vi "Dyson_X682_Attachment_Provisioning_Tester_Ver 1.0.0.0.vi"() -> ()   [LabVIEW 2017]
uses:
  Ctrls/MainStep.ctl
  Ctrls/AllControls.ctl
  <vilib>/Utility/miscctls.llb/LVRowAndColumnTypeDef.ctl
  ComVIS/Files/Ini/WriteIniFiles_ByVarient.vi
panel:
  in  "Recipe":string(combo)
  in  "MES Status":bool
  in  "maintenance":bool
  in  "mode":enum32{"Production mode", "Engineering mode"}(tab)
  out "Fail resume":bool caption="TotalResult"
  out "Table":string[][](table)
  out "LogInfo":string caption="Log"
  in  "AlarmData":i32(listbox)=-1
  out "Device state":bool caption="TotalResult"
  out "CT":dbl format="%#_3f"
  in  "ProductID:":string
  in  "TestInfo":T1 {"Yield" format="%#_g%"}
  out "MES_Status":string
  out "TestMode":string
  in  "Stop":bool
  in  "Start":bool
  in  "Exit":bool
  in  "Login":bool
  out "Login_status":string="Operator:Operator"
  out "OpenStatus":string
  in  "error in (no error)":errorcluster caption="错误输入（无错误）"
  # "Dyson X682 Attachment Provisioning Tester  v1.0.0.0"
  # "Waiting Barcode scanning"
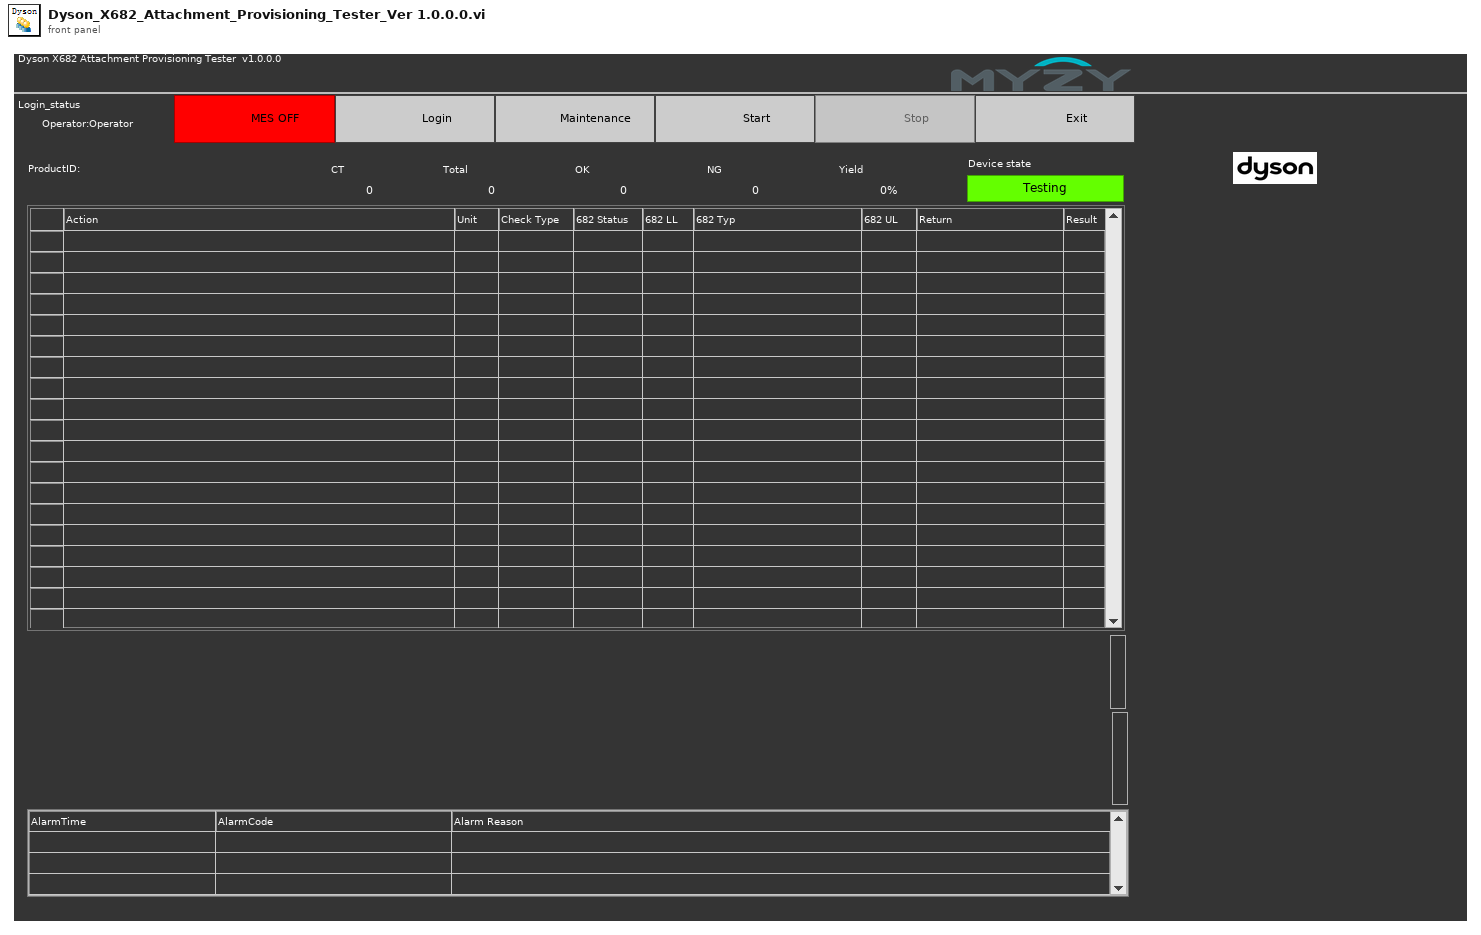
[diagram p1: front panel]
types:
  T1 = cluster{"Total":i32, "OK":i32, "NG":i32, "Yield":dbl}
  T2 = typedef "MainStep.ctl" = enum16{"Initialize", "ReadAllFiles", "ResetHardware", "Run", "Exit"}
  T3 = typedef "AllControls.ctl" = cluster{"MainVI":refnum<vi>, "AlarmInfo":refnum<vi>, "Log":refnum<vi>, "Current CT":refnum<vi>, "ProductID":refnum<vi>, "Device state":refnum<vi>, "MES":refnum<vi>, "mode":refnum<vi>, "TestInfo":refnum<vi>, "SubPnl":refnum<vi>, "Table":refnum<vi>, "MES bool":refnum<vi>, "TestMode":refnum<vi>, "Recipe":refnum<vi>, "Fail resume":refnum<vi>, "LogIn":refnum<vi>, "Start":refnum<vi>, "Maintenance":refnum<vi>, "Stop":refnum<vi>, "Exit":refnum<vi>}
  T4 = enum32{"Invalid", "Standard", "Closed", "Hidden", "Minimized", "Maximized"}
  T5 = enum16{"Ini", "Standby", "Running", "Engineering"}
  T6 = typedef "LVRowAndColumnTypeDef.ctl" = cluster{"Row":i32, "Column":i32}
  T7 = enum32{"invalid app kind", "Development System", "Run Time System", "Student Edition", "Embedded LabVIEW", "Evaluation", "Custom"}
  T8 = typedef "amc_Message Queue.ctl" = refnum<queue>
  T9 = typedef "HD Config.ctl" = cluster{" PC":cluster{"PC Address":u8[], "PC Port":i32}, "FCO":cluster{"COM":refnum<visa-resource-name>, "Baudrate":u32}, "DC Power ":cluster{"COM":refnum<visa-resource-name>, "Baudrate":u32}, "PW3336":cluster{"COM":refnum<visa-resource-name>, "Baudrate":u32}, "Lefoo":cluster{"COM":refnum<visa-resource-name>, "Baudrate":u32}, "AI Model":cluster{"COM":refnum<visa-resource-name>, "Baudrate":u32}, "DIPC":cluster{"COM":refnum<visa-resource-name>}, "RFID":cluster{"IP Address":string, "Port":u16, "Retry":u16}, "Motor":cluster{"COM":refnum<visa-resource-name>, "Baudrate":u32}, "Fail_resume_mode":bool, "GRR":bool}
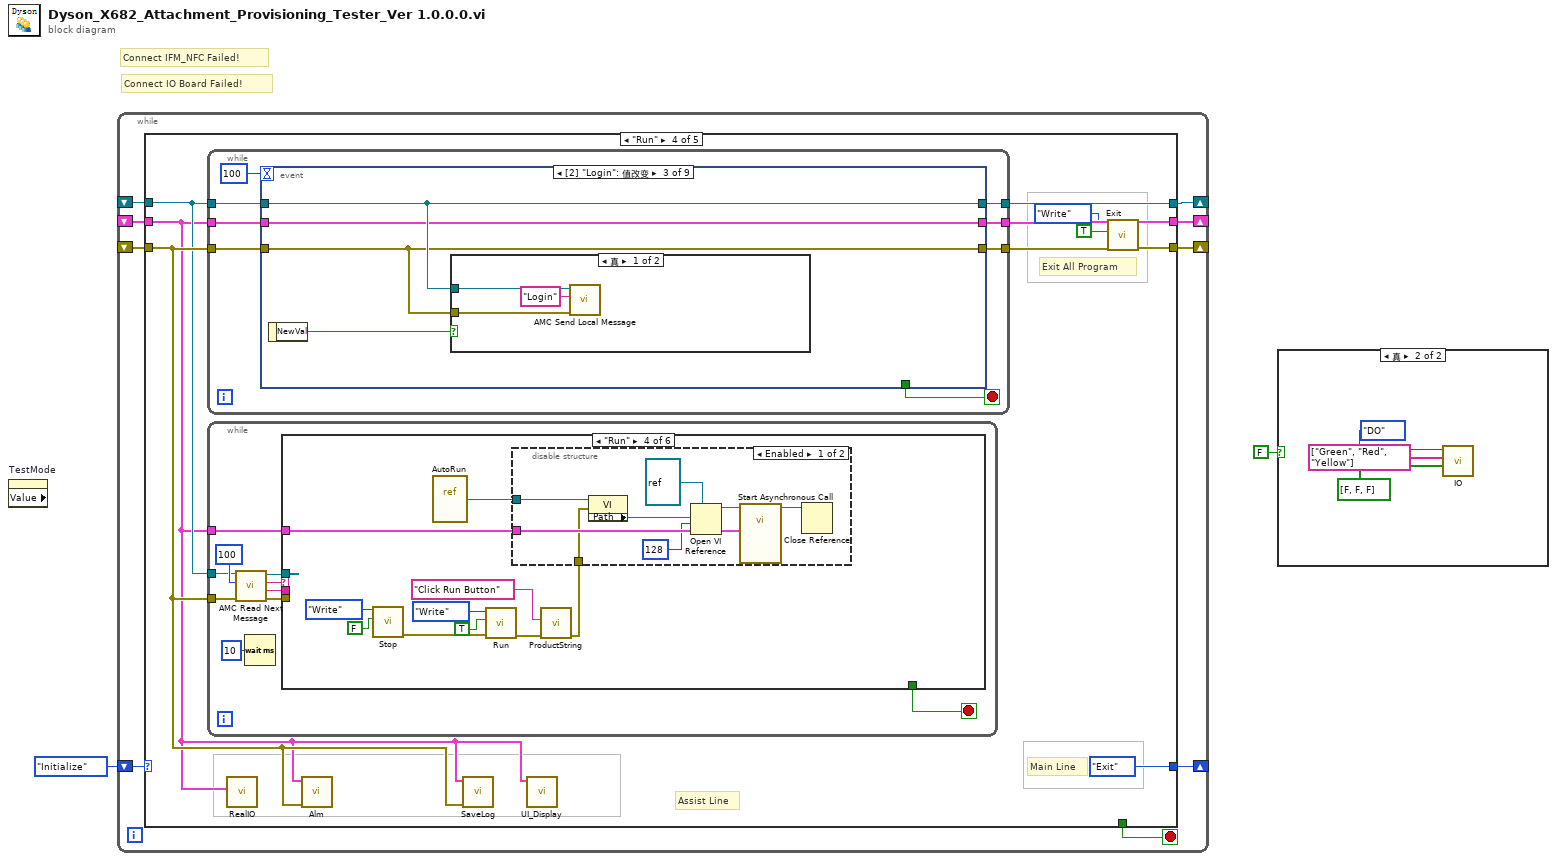
[diagram p0: block diagram]
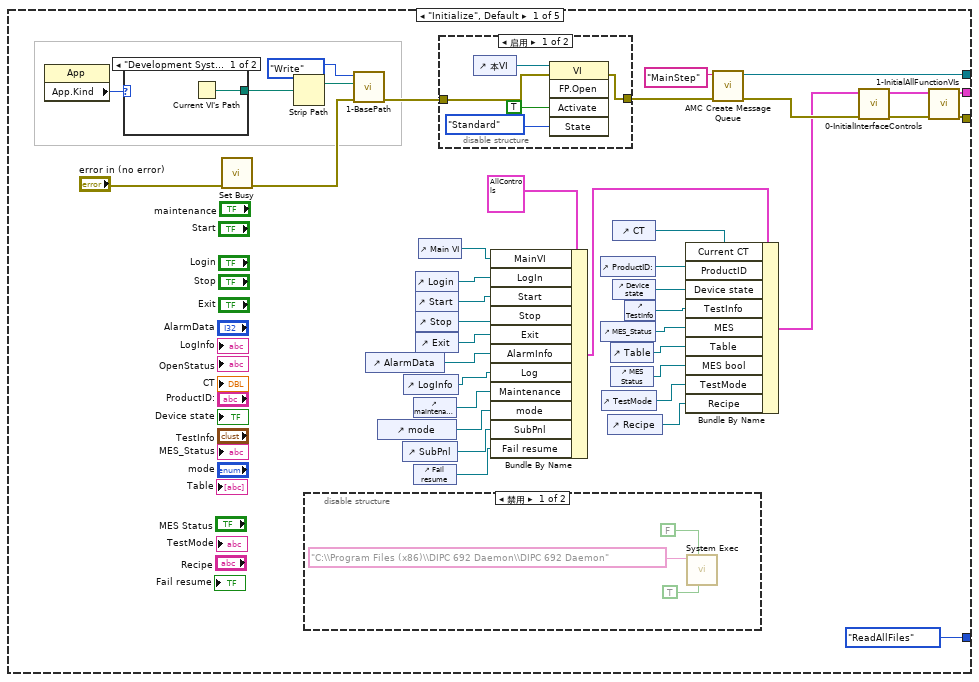
[diagram p3: hidden frame]
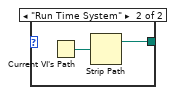
[diagram p6: hidden frame]
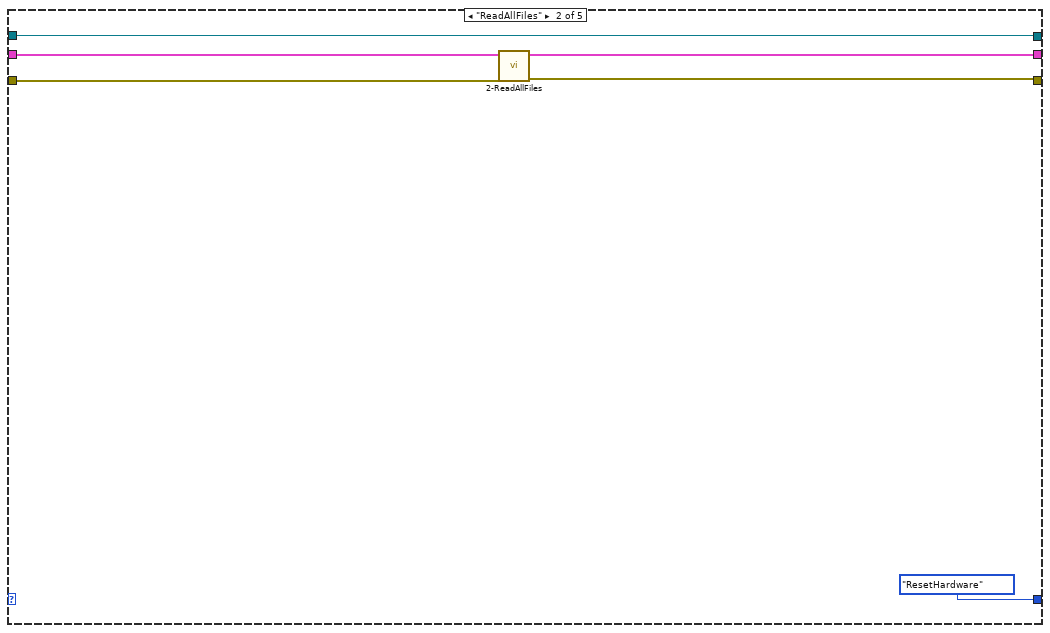
[diagram p7: hidden frame]
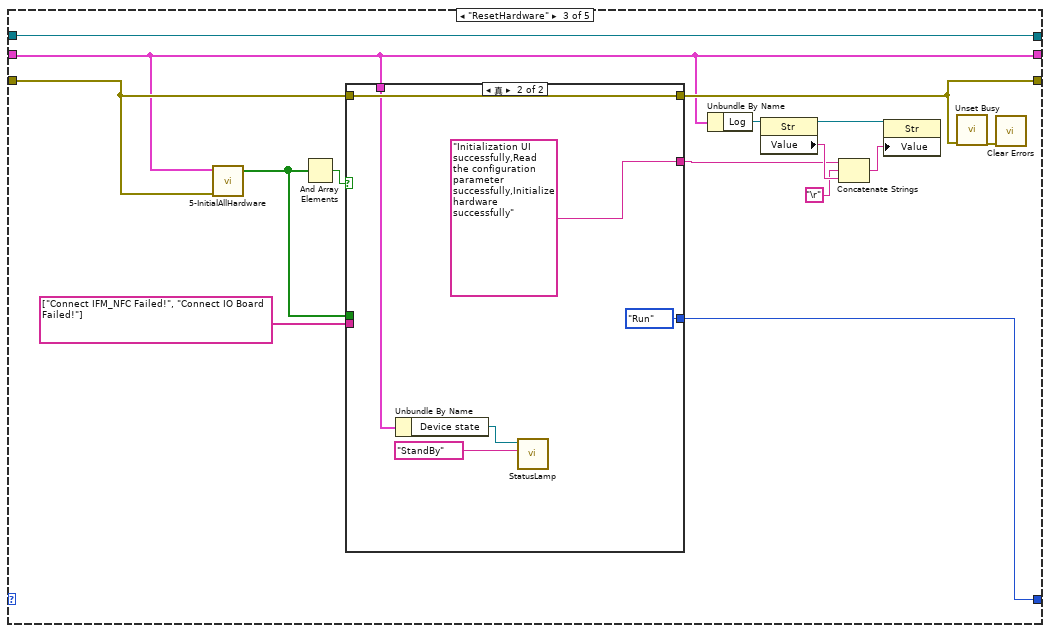
[diagram p8: hidden frame]
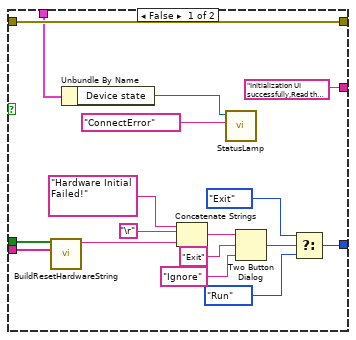
[diagram p9: hidden frame]
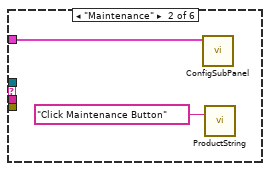
[diagram p11: hidden frame]
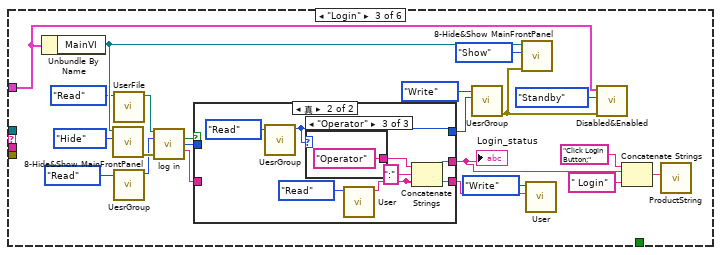
[diagram p12: hidden frame]
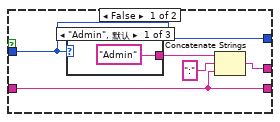
[diagram p13: hidden frame]
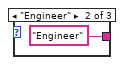
[diagram p14: hidden frame]
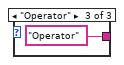
[diagram p15: hidden frame]
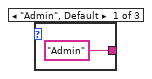
[diagram p16: hidden frame]
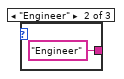
[diagram p17: hidden frame]
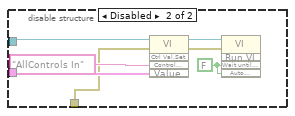
[diagram p18: hidden frame]
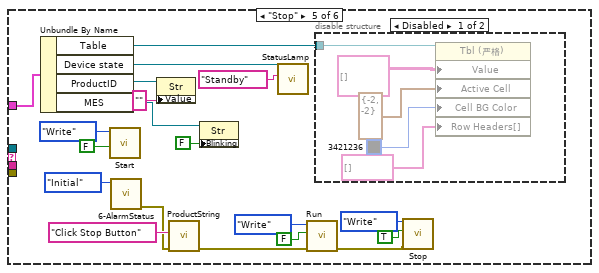
[diagram p19: hidden frame]
diagram:
  # "Connect IO Board Failed!"
  # "Connect IFM_NFC Failed!"
  n1 = property on="TestMode" class="Str" props=["Value"]() -> ()  [unwired: 2 in, 3 out]
  n2 = while {
    shift-right: [w10] -> _
    shift-left: MainStep."Initialize" -> [w11]
    shift-right: [w8] -> _
    shift-left: _ -> [w3]
    shift-right: [w6] -> _
    shift-left: _ -> [w4]
    shift-right: [w7] -> _
    shift-left: _ -> [w5]
    stop <- w9 stop-if-true
    n3 = case shown="\"Run\"" w11 {
      tunnel: [MainStep."ReadAllFiles" MainStep."ResetHardware" w83 MainStep."Exit" MainStep."Exit"] -> w10
      tunnel: [_ _ _ _ TRUE] -> w9
      tunnel: [w38 w63 w78 w110 w347] -> w8
      tunnel: [w46 w67 w82 w115 _] -> w7
      tunnel: [w39 w65 w76 w114 w345] -> w6
      tunnel: w5 -> [_ w67 w82 w108 w348]
      tunnel: w4 -> [_ w66 w76 w107 w345]
      tunnel: w3 -> [_ w64 w79 w109 w346]
      frame "Initialize", Default {
        n4 = property class="App"() -> ("App.Kind"=w50:T7)  [unwired: 2 in, 2 out]
        n5 = case shown="\"Development System\", 默认" w50 {
          tunnel: [w60 w61] -> w49
          frame "Development System", Default {
            n6 = Current VI's Path() -> (path=w60:path)
          }
          frame "Run Time System" {
            n7 = Current VI's Path() -> (path=w62:path)
            n8 = Strip Path(path=w62) -> (stripped path=w61:path)  [unwired: 1 out]
          }
        }
        n9 = call <vilib>:"Set Busy.vi"("error in (no error)"="error in (no error)") -> ("error out"=w18:errorcluster)  [unwired: 9 in, 1 out]
        n10 = Strip Path(path=w49) -> (stripped path=w19:path)  [unwired: 1 out]
        n11 = disable-structure shown="禁用" {
          frame Disabled {
            n12 = call <vilib>:"System Exec.vi"("run minimized? (F)"=TRUE, "wait until completion? (T)"=FALSE, "command line"="C:\\Program Files (x86)\\DIPC 692 Daemon\\DIPC 692 Daemon") -> ()  [unwired: 5 in, 4 out]
          }
          frame Enabled {
          }
        }
        n13 = call "1-BasePath.vi"("error in (no error)"=w18, "Path In"=w19, "Step"=enum16{"Initial", "Write", "Read"}."Write") -> ("error out"=w17:errorcluster)  [unwired: 7 in, 1 out]
        n14 = control-ref of="AlarmData"() -> (w44:refnum<vi>)
        n15 = control-ref of="mode"() -> (w25:refnum<vi>)
        n16 = control-ref of="SubPnl"() -> (w23:refnum<vi>)
        n17 = control-ref of="LogInfo"() -> (w43:refnum<vi>)
        n18 = control-ref of="maintenance"() -> (w24:refnum<vi>)
        n19 = control-ref of="Fail resume"() -> (w13:refnum<vi>)
        n20 = control-ref of="Login"() -> (w26:refnum<vi>)
        n21 = control-ref of="Start"() -> (w27:refnum<vi>)
        n22 = control-ref of="Stop"() -> (w28:refnum<vi>)
        n23 = control-ref of="Exit"() -> (w29:refnum<vi>)
        n24 = control-ref of="Main VI"() -> (w36:refnum<vi>)
        n25 = disable-structure shown="启用" {
          disable-tunnel: w17 -> [w56 w59]
          disable-tunnel: [w54 w59] -> w47
          frame Enabled {
            n26 = control-ref of="本VI"() -> (w58:refnum<vi>)
            n27 = invoke class="VI" method="FP.Open"(reference=w58, error in=w56, "Activate"=TRUE ("激活？"), "State"=T4."Standard" ("状态")) -> (error out=w54:errorcluster)  [unwired: 1 in, 4 out]
          }
          frame Disabled {
          }
        }
        n28 = Bundle By Name(cluster=T3 {"MainVI"=refnum, "AlarmInfo"=refnum, "Log"=refnum, "Current CT"=refnum, "ProductID"=refnum, "Device state"=refnum, "MES"=refnum, "mode"=refnum, "TestInfo"=refnum, "SubPnl"=refnum, "Table"=refnum, "MES bool"=refnum, "TestMode"=refnum, "Recipe"=refnum, "Fail resume"=refnum, "LogIn"=refnum, "Start"=refnum, "Maintenance"=refnum, "Stop"=refnum, "Exit"=refnum}, "MainVI"=w36, "LogIn"=w26, "Start"=w27, "Stop"=w28, "Exit"=w29, "AlarmInfo"=w44, "Log"=w43, "Maintenance"=w24, "mode"=w25, "SubPnl"=w23, "Fail resume"=w13) -> (w35:T3)
        n29 = control-ref of="ProductID:"() -> (w33:refnum<vi>)
        n30 = control-ref of="MES_Status"() -> (w30:refnum<vi>)
        n31 = control-ref of="TestMode"() -> (w15:refnum<vi>)
        n32 = control-ref of="Recipe"() -> (w14:refnum<vi>)
        n33 = control-ref of="Table"() -> (w21:refnum<vi>)
        n34 = control-ref of="MES Status"() -> (w16:refnum<vi>)
        n35 = control-ref of="CT"() -> (w32:refnum<vi>)
        n36 = control-ref of="Device state"() -> (w34:refnum<vi>)
        n37 = control-ref of="TestInfo"() -> (w31:refnum<vi>)
        n38 = Bundle By Name(cluster=w35, "Current CT"=w32, "ProductID"=w33, "Device state"=w34, "TestInfo"=w31, "MES"=w30, "Table"=w21, "MES bool"=w16, "TestMode"=w15, "Recipe"=w14) -> (w22:T3)
        n39 = call "AMC Create Message Queue.vi"("error in (no error)"=w47, "Message Queue Name"="MainStep" ("Message queue name (unnamed)")) -> ("error out"=w42:errorcluster, "Message Queue out"=w46:T8)  [unwired: 3 in, 5 out]
        n40 = call "0-InitialInterfaceControls.vi"("error in (no error)"=w42, "AllControls IN"=w22) -> ("error out"=w41:errorcluster, "AllControls Out"=w40:T3)  [unwired: 8 in]
        n41 = call "1-InitialAllFunctionVIs.vi"("error in (no error)"=w41, "AllControls IN"=w40) -> ("error out"=w38:errorcluster, "AllControls Out"=w39:T3)  [unwired: 8 in]
      }
      frame "ReadAllFiles" {
        n42 = call "2-ReadAllFiles.vi"("error in (no error)"=w64, "AllControls IN"=w66) -> ("error out"=w63:errorcluster, "AllControls Out"=w65:T3)  [unwired: 8 in]
      }
      frame "ResetHardware" {
        n43 = call "5-InitialAllHardware.vi"("error in (no error)"=w79, "AllControls IN"=w76) -> ("InitalResult"=w69:bool[])  [unwired: 9 in]
        n44 = And Array Elements(Boolean array=w69) -> (logical AND=w81:bool)
        n45 = case shown="真" w81 {
          tunnel: [w91 MainStep."Run"] -> w83
          tunnel: w79 -> [w100 w105]
          tunnel: string[] ["Connect IFM_NFC Failed!", "Connect IO Board Failed!"] -> [w89 _]
          tunnel: w69 -> [w90 _]
          tunnel: [w100 w105] -> w78
          tunnel: ["Initialization UI successfully,Read the configuration parameter successfully,Initialize hardware failure" ("值") "Initialization UI successfully,Read the configuration parameter successfully,Initialize hardware successfully" ("值")] -> w72
          tunnel: w76 -> [w84 w103]
          frame False {
            n46 = call "BuildResetHardwareString.vi"("String"=w89, "Error"=w90) -> ("DataOut"=w88:string)  [unwired: 9 in]
            n47 = Unbundle By Name(w84) -> ("Device state"=w85:refnum<vi>)
            n48 = Concatenate Strings("Hardware Initial Failed!" ("caption"), "\r", w88) -> (w98:string)
            n49 = call "StatusLamp.vi"("State"="ConnectError", "Boolean输入"=w85) -> ()  [unwired: 9 in, 1 out]
            n50 = Two Button Dialog(message=w98, 1:"Ignore" ("F按钮名称（“取消”）"), 2:"Exit" ("T按钮名称（“确定”）")) -> (T button?=w94:bool)
            n51 = Select(t=MainStep."Exit", s=w94, f=MainStep."Run") -> (s? t:f=w91:T2)
          }
          frame True {
            n52 = Unbundle By Name(w103) -> ("Device state"=w101:refnum<vi>)
            n53 = call "StatusLamp.vi"("State"="StandBy", "Boolean输入"=w101) -> ()  [unwired: 9 in, 1 out]
          }
        }
        n54 = Unbundle By Name(w76) -> ("Log"=w73:refnum<vi>)
        n55 = property class="Str"(reference=w73) -> (reference out=w71:refnum<vi>, "Value"=w75:string)  [unwired: 1 in, 1 out]
        n56 = Concatenate Strings(w72, "\r", w75) -> (w70:string)
        n57 = property class="Str"(reference=w71, "Value"=w70) -> ()  [unwired: 1 in, 2 out]
        n58 = call <vilib>:"Unset Busy.vi"("error in (no error)"=w78) -> ("error out"=w77:errorcluster)  [unwired: 10 in]
        n59 = call <vilib>:"Clear Errors.vi"("error in (no error)"=w77) -> ()  [unwired: 5 in, 2 out]
      }
      frame "Run" {
        # "Exit All Program"
        # "Assist Line"
        # "Main Line"
        n60 = while {
          tunnel: w108 -> [w227]
          tunnel: w107 -> [w226]
          tunnel: w109 -> [w225]
          tunnel: [w224] -> w115
          tunnel: [w223] -> w114
          tunnel: [w222] -> w111
          stop <- w221 stop-if-true
          n61 = event shown="[2] \"Login\": 值改变" {
            selector: _ -> [_ _ _ _ _ _ _ _ _]
            dyn-events: _ -> [_ _ _ _ _ _ _ _ _]
            timeout: 100 -> [_ _ _ _ _ _ _ _ _]
            tunnel: w227 -> [w230 w238 w263 w269 w281 w306 w320 w329 w336]
            tunnel: w226 -> [w229 w233 w261 w268 w279 w304 w318 w331 w341]
            tunnel: w225 -> [w228 w237 w262 w271 w280 w305 w319 w328 w337]
            tunnel: [w230 w238 w263 w269 w281 w306 w320 w329 w336] -> w224
            tunnel: [w229 w233 w261 w268 w279 w304 w318 w331 w341] -> w223
            tunnel: [w228 w237 w262 w271 w280 w305 w319 w328 w337] -> w222
            tunnel: [_ _ _ _ _ _ _ w327 w340] -> w221
            event Timeout {
              n62 = event-data() -> ()  [unwired: 1 in, 1 out]
            }
            event "Recipe": Value Change {
              n63 = event-data() -> ("OldVal"=w236:string, "NewVal"=w234:string)  [unwired: 1 in]
              n64 = Not Equal?(x=w236, y=w234) -> (x != y?=w235:bool)
              n65 = call "Run.vi"("Step"=enum16{"Initial", "Write", "Read"}."Read") -> ("Run Out"=w231:bool)  [unwired: 9 in, 1 out]
              n66 = case shown="假" w231 {
                tunnel: w235 -> [w241 _]
                tunnel: w234 -> [w240 _]
                tunnel: w233 -> [w239 _]
                frame False {
                  n67 = case shown="真" w241 {
                    tunnel: w240 -> [_ w255]
                    tunnel: w239 -> [_ w243]
                    frame False {
                    }
                    frame True {
                      w256 = cluster{"Recipe":string} {"Recipe"=""}  # Recipe
                      n68 = call "1-BasePath.vi"("Step"=enum16{"Initial", "Write", "Read"}."Read") -> ("Path Out"=w257:path)  [unwired: 9 in, 1 out]
                      n69 = call "ReadConfigandSetting.vi"("Recipe"=w255, "Path Out"=w257) -> ("TableData"=w244:string[][])  [unwired: 7 in, 2 out]
                      n70 = Bundle By Name(cluster=w256, "Recipe"=w255) -> (w254:cluster{"Recipe":string})
                      n71 = Build Path(base path=w257, name or relative path="data\\Recipe.ini") -> (appended path=w259:path)
                      n72 = Unbundle By Name(w243) -> ("Table"=w242:refnum<vi>)
                      n73 = call-poly "Read&WriteFile.vi"("Variant"=w254, "path"=w259) -> ()  [unwired: 9 in, 1 out]
                      n74 = Delete From Array(array=w244, length=1 ("长度"), index (row)=0 ("索引 (行)")) -> (deleted portion=w252:string[][], array with subset deleted=w250:string[][])  [unwired: 1 in]
                      n75 = call "Select_UUT_Table.vi"("all Title"=w252, "all Table"=w250) -> ("Title"=w251:string[], "Table"=w253:string[][])  [unwired: 8 in]
                      n76 = property class="Tbl (严格)"(reference=w242, "Value"=w253, "Column Headers[]"=w251, "Active Cell"=T6 {"Row"=-2, "Column"=-2} ("活动单元格:活动单元格"), "Cell BG Color"=u32 3421236, "Row Headers[]"=string[] [] ("Row Header Strings[]")) -> ()  [unwired: 1 in, 2 out]
                    }
                  }
                }
                frame True {
                }
              }
            }
            event "Login": Value Change {
              n77 = event-data() -> ("NewVal"=w264:bool)  [unwired: 1 in]
              n78 = case shown="真" w264 {
                tunnel: w263 -> [w267 _]
                tunnel: w262 -> [w266 _]
                frame True {
                  n79 = call "AMC Send Local Message.vi"("error in (no error)"=w266, "Message Name"="Login", "Message Queue in"=w267) -> ()  [unwired: 7 in, 2 out]
                }
                frame False {
                }
              }
            }
            event "maintenance": Value Change {
              n80 = event-data() -> ("NewVal"=w272:bool)  [unwired: 1 in]
              n81 = Unbundle By Name(w268) -> ("mode"=w270:refnum<vi>)
              n82 = case shown="真" w272 {
                tunnel: w270 -> [w278 _]
                tunnel: w269 -> [w275 _]
                tunnel: w268 -> [w274 _]
                frame True {
                  n83 = call "AMC Send Local Message.vi"("Message Name"="Maintenance", "Message Queue in"=w275) -> ()  [unwired: 8 in, 2 out]
                  n84 = property class="TabCtl (严格)"(reference=w278, "Value"=enum32{"Production mode", "Engineering mode"}."Engineering mode" ("值")) -> ()  [unwired: 1 in, 2 out]
                  n85 = call "Disabled&Enabled.vi"("Mode in"=T5."Engineering", "AllControls In"=w274) -> ()  [unwired: 9 in, 1 out]
                }
                frame False {
                }
              }
            }
            event "Start": Value Change {
              n86 = event-data() -> ("NewVal"=w282:bool)  [unwired: 1 in]
              n87 = case shown="真" w282 {
                tunnel: w281 -> [w287 _]
                tunnel: w280 -> [w286 _]
                tunnel: w279 -> [w283 _]
                frame True {
                  n88 = call "AMC Send Local Message.vi"("error in (no error)"=w286, "Message Name"="Run", "Message Queue in"=w287) -> ()  [unwired: 7 in, 2 out]
                  n89 = call "Disabled&Enabled.vi"("Mode in"=T5."Running", "AllControls In"=w283) -> ()  [unwired: 9 in, 1 out]
                }
                frame False {
                }
              }
            }
            event "MES Status": Value Change {
              n90 = event-data() -> ("NewVal"=w289:bool)  [unwired: 1 in]
              n91 = Unbundle By Name(w304) -> ("MES bool"=w297:refnum<vi>, "TestMode"=w288:refnum<vi>)
              n92 = call "HD_Config.vi"("Step"=enum16{"Initial", "Write", "Read"}."Read") -> ("HD Config out"=w296:T9)  [unwired: 9 in, 1 out]
              n93 = Unbundle By Name(w296) -> ("Fail_resume_mode"=w293:bool, "GRR"=w291:bool)
              n94 = Not(x=w289) -> (.not. x?=w295:bool)
              n95 = Or(x=w293, y=w295) -> (x .or. y?=w294:bool)
              n96 = case shown="假" w291 {
                tunnel: w294 -> [w308 _]
                tunnel: [w307 "GRR"] -> w292
                frame False {
                  n97 = case shown="真" w308 {
                    tunnel: ["Production" "Engineering"] -> w307
                    frame False {
                    }
                    frame True {
                    }
                  }
                }
                frame True {
                }
              }
              n98 = property class="Str"(reference=w288, "Value"=w292) -> ()  [unwired: 1 in, 2 out]
              n99 = Select(t="MES ON", s=w289, f="MES OFF") -> (s? t:f=w298:string)
              n100 = case shown="\"MES ON\", 默认" w298 {
                selector: w298 -> [w312 w315]
                tunnel: [TRUE FALSE] -> w300
                tunnel: [w312 w315] -> w301
                tunnel: [cluster{u32, u32}[] [{6618880, 6618880}] cluster{u32, u32}[] [{16711680, 16711680}]] -> w299
                frame "MES ON", Default {
                }
                frame "MES OFF" {
                }
              }
              n101 = property on="属性节点" class="Bool (严格)"(reference=w297, "Value"=w300, "Colors [4]"=w299, "BoolText.Text"=w301) -> ()  [unwired: 1 in, 2 out]
            }
            event "Stop": Value Change {
              n102 = event-data() -> ("NewVal"=w321:bool)  [unwired: 1 in]
              n103 = case shown="真" w321 {
                tunnel: w320 -> [w326 _]
                tunnel: w319 -> [w325 _]
                tunnel: w318 -> [w322 _]
                frame True {
                  n104 = call "AMC Send Local Message.vi"("error in (no error)"=w325, "Message Name"="Stop", "Message Queue in"=w326) -> ()  [unwired: 7 in, 2 out]
                  n105 = call "Disabled&Enabled.vi"("Mode in"=T5."Standby", "AllControls In"=w322) -> ()  [unwired: 9 in, 1 out]
                }
                frame False {
                }
              }
            }
            event "Exit": Value Change {
              n106 = event-data() -> ("NewVal"=w330:bool)  [unwired: 1 in]
              n107 = case shown="真" w330 {
                tunnel: w329 -> [_ w335]
                tunnel: w328 -> [_ w334]
                tunnel: [_ TRUE] -> w327
                frame False {
                }
                frame True {
                  n108 = call "AMC Send Local Message.vi"("error in (no error)"=w334, "Message Name"="Exit", "Message Queue in"=w335) -> ()  [unwired: 7 in, 2 out]
                }
              }
            }
            event Panel Close? {
              n109 = event-data() -> ()  [unwired: 1 in, 1 out]
              n110 = Two Button Dialog(message="Are you sure to Exit system?") -> (T button?=w339:bool)  [unwired: 2 in]
              n111 = case shown="假" w339 {
                selector: w339 -> [w343 w344]
                tunnel: [w343 w344] -> w340
                frame False {
                }
                frame True {
                }
              }
              n112 = Not(x=w340) -> (.not. x?=w342:bool)
              n113 = event-data("Discard?"=w342) -> ()  [unwired: 1 in, 1 out]
            }
          }
        }
        n114 = while {
          tunnel: w107 -> [w126]
          tunnel: w109 -> [w123]
          tunnel: w108 -> [w120]
          stop <- w117 stop-if-true
          n115 = call "AMC Read Next Message.vi"("error in (no error)"=w123, "timeout (1ms)"=100 ("Timeout"), "Message Queue in"=w120) -> ("error out"=w122:errorcluster, "Message Value"=w118:string, "Message Name"=w121:string, "Message Queue out"=w119:T8)  [unwired: 1 in, 4 out]
          n116 = Wait (ms)(milliseconds to wait=u32 10 ("毫秒倍数")) -> ()  [unwired: 1 out]
          n117 = case shown="\"Run\"" w121 {
            tunnel: w126 -> [_ w128 w136 w171 w211 _]
            tunnel: w122 -> [_ _ _ _ _ _]
            tunnel: [_ _ _ _ _ TRUE] -> w117
            tunnel: w119 -> [_ _ _ _ _ _]
            tunnel: w118 -> [_ _ _ _ _ _]
            frame "Null", Default {
            }
            frame "Maintenance" {
              n118 = call "ConfigSubPanel.vi"("AllControls"=w128) -> ()  [unwired: 11 in]
              n119 = call "ProductString.vi"("String"="Click Maintenance Button" ("值")) -> ()  [unwired: 10 in, 1 out]
            }
            frame "Login" {
              n120 = Unbundle By Name(w136) -> ("MainVI"=w149:refnum<vi>)
              n121 = call "8-Hide&Show MainFrontPanel.vi"("Hide&Show"=enum16{"Hide", "Show"}."Hide", "This VI"=w149) -> ("error out"=w147:errorcluster)  [unwired: 9 in]
              n122 = call "UserFile.vi"("Step"=enum16{"Initial", "Write", "Read"}."Read") -> ("UserPath out"=w146:path)  [unwired: 9 in, 1 out]
              n123 = call "UesrGroup.vi"("Step"=enum16{"Initial", "Write", "Read"}."Read") -> ("User group out"=w129:enum16{"Operator", "Engineer", "Admin"})  [unwired: 9 in, 1 out]
              n124 = call "log in.vi"("路径"=w146, "UserGroups in"=w129, "error in (no error)"=w147) -> ("Giveup?"=w144:bool, "UserGroups"=w143:enum16{"Operator", "Engineer", "Admin"}, "User"=w142:string)  [unwired: 8 in, 2 out]
              n125 = case shown="真" w144 {
                tunnel: [w152 w159] -> w138
                tunnel: [w153 w163] -> w132
                tunnel: [w151 w161] -> w140
                tunnel: w143 -> [w151 _]
                tunnel: w142 -> [w152 _]
                frame False {
                  n126 = case shown="\"Admin\", 默认" w151 {
                    tunnel: ["Admin" "Engineer" "Operator"] -> w155
                    frame "Admin", Default {
                    }
                    frame "Engineer" {
                    }
                    frame "Operator" {
                    }
                  }
                  n127 = Concatenate Strings(w155, ":" ("字符串"), w152) -> (w153:string)
                }
                frame True {
                  n128 = call "UesrGroup.vi"("Step"=enum16{"Initial", "Write", "Read"}."Read") -> ("User group out"=w161:enum16{"Operator", "Engineer", "Admin"})  [unwired: 9 in, 1 out]
                  n129 = case shown="\"Operator\"" w161 {
                    tunnel: ["Admin" "Engineer" "Operator"] -> w165
                    frame "Admin", Default {
                    }
                    frame "Engineer" {
                    }
                    frame "Operator" {
                    }
                  }
                  n130 = call "User.vi"("Step"=enum16{"Initial", "Write", "Read"}."Read") -> ("User out"=w159:string)  [unwired: 9 in, 1 out]
                  n131 = Concatenate Strings(w165, ":" ("字符串"), w159) -> (w163:string)
                }
              }
              "Login_status" <- w132
              n132 = call "UesrGroup.vi"("User group in"=w140, "Step"=enum16{"Initial", "Write", "Read"}."Write") -> ("错误输出"=w135:errorcluster)  [unwired: 8 in, 1 out]
              n133 = call "8-Hide&Show MainFrontPanel.vi"("error in (no error)"=w135, "Hide&Show"=enum16{"Hide", "Show"}."Show", "This VI"=w149) -> ()  [unwired: 8 in, 1 out]
              n134 = call "User.vi"("User in"=w138, "Step"=enum16{"Initial", "Write", "Read"}."Write") -> ()  [unwired: 8 in, 2 out]
              n135 = call "Disabled&Enabled.vi"("error in (no error)"=w135, "Mode in"=T5."Standby", "AllControls In"=w136) -> ()  [unwired: 8 in, 1 out]
              n136 = Concatenate Strings("Click Login Button;" ("String"), w132, " Login" ("字符串")) -> (w133:string)
              n137 = call "ProductString.vi"("String"=w133) -> ()  [unwired: 10 in, 1 out]
            }
            frame "Run" {
              n138 = call "Stop.vi"("Stop In"=FALSE ("AutoStopping In"), "Step"=enum16{"Initial", "Write", "Read"}."Write") -> ("error out"=w177:errorcluster)  [unwired: 8 in, 1 out]
              n139 = vi-ref "AutoRun.vi"() -> (w169:refnum<vi>)
              n140 = call "Run.vi"("error in (no error)"=w177, "Run In"=TRUE ("AutoRun In"), "Step"=enum16{"Initial", "Write", "Read"}."Write") -> ("error out"=w172:errorcluster)  [unwired: 7 in, 1 out]
              n141 = call "ProductString.vi"("error"=w172, "String"="Click Run Button" ("值")) -> ("error  out"=w170:errorcluster)  [unwired: 9 in]
              n142 = disable-structure shown="Enabled" {
                disable-tunnel: w171 -> [w183 w189]
                disable-tunnel: w170 -> [w181 w187]
                disable-tunnel: w169 -> [w180 w188]
                frame Enabled {
                  n143 = property class="VI"(reference=w180, error in=w181) -> ("Path"=w186:path)  [unwired: 2 out]
                  n144 = Open VI Reference(type specifier VI Refnum (for type only)=refnum<vi> refnum ("application reference (local)"), vi path=w186, options=128) -> (vi reference=w184:refnum<vi>)  [unwired: 3 in, 1 out]
                  n145 = call-by-ref "Start Asynchronous Call"(reference=w184, "AllControls In"=w183) -> (reference out=w182:refnum<vi>)  [unwired: 12 in, 1 out]
                  n146 = Close Reference(reference=w182) -> ()  [unwired: 1 in, 1 out]
                }
                frame Disabled {
                  w190 = FALSE ("Wait Until Done")
                  n147 = invoke class="VI" method="Ctrl Val.Set"(reference=w188, error in=w187, "Control Name"="AllControls In", "Value"=w189) -> (reference out=w192:refnum<vi>, error out=w193:errorcluster)  [unwired: 1 in, 3 out]
                  n148 = invoke class="VI" method="Run VI"(reference=w192, error in=w193, "Wait until done"=w190, "Auto Dispose Ref"=w190) -> ()  [unwired: 1 in, 5 out]
                }
              }
            }
            frame "Stop" {
              n149 = Unbundle By Name(w211) -> ("Table"=w205:refnum<vi>, "Device state"=w208:refnum<vi>, "ProductID"=w210:refnum<vi>, "MES"=w203:refnum<vi>)
              n150 = call "Start.vi"("Start In"=FALSE, "Step"=enum16{"Initial", "Write", "Read"}."Write") -> ()  [unwired: 8 in, 2 out]
              n151 = call "6-AlarmStatus.vi"("Step"=enum16{"Initial", "Write", "Read"}."Initial") -> ("error out"=w204:errorcluster)  [unwired: 9 in, 1 out]
              n152 = property class="Str"(reference=w210, "Value"="") -> ()  [unwired: 1 in, 2 out]
              n153 = call "ProductString.vi"("error"=w204, "String"="Click Stop Button" ("值")) -> ("error  out"=w206:errorcluster)  [unwired: 9 in]
              n154 = property class="Str"(reference=w203, "Blinking"=FALSE ("闪烁")) -> ()  [unwired: 1 in, 2 out]
              n155 = call "StatusLamp.vi"("State"="Standby", "Boolean输入"=w208) -> ()  [unwired: 9 in, 1 out]
              n156 = call "Run.vi"("error in (no error)"=w206, "Run In"=FALSE ("AutoRun In"), "Step"=enum16{"Initial", "Write", "Read"}."Write") -> ("error out"=w201:errorcluster)  [unwired: 7 in, 1 out]
              n157 = disable-structure shown="Disabled" {
                disable-tunnel: w205 -> [w214 _]
                frame Disabled {
                  n158 = property class="Tbl (严格)"(reference=w214, "Value"=string[][] [] ("值"), "Active Cell"=T6 {"Row"=-2, "Column"=-2} ("活动单元格:活动单元格"), "Cell BG Color"=u32 3421236, "Row Headers[]"=string[] [] ("Row Header Strings[]")) -> ()  [unwired: 1 in, 2 out]
                }
                frame Enabled {
                }
              }
              n159 = call "Stop.vi"("error in (no error)"=w201, "Stop In"=TRUE ("AutoStopping In"), "Step"=enum16{"Initial", "Write", "Read"}."Write") -> ()  [unwired: 7 in, 2 out]
            }
            frame "Exit" {
              n160 = call "ProductString.vi"("String"="Click Exit Button" ("值")) -> ()  [unwired: 10 in, 1 out]
            }
          }
        }
        n161 = call "RealIO.vi"("AllControls Out"=w107) -> ()  [unwired: 11 in]
        n162 = call "Alm.vi"("error in (no error)"=w109, "AllControls Out"=w107) -> ()  [unwired: 10 in]
        n163 = call "SaveLog.vi"("错误输入（无错误）"=w109, "AllControls In"=w107) -> ()  [unwired: 9 in, 1 out]
        n164 = call "UI_Display.vi"("AllControls In"=w107) -> ()  [unwired: 11 in]
        n165 = call "Exit.vi"("error in (no error)"=w111, "Exit In"=TRUE, "Step"=enum16{"Initial", "Write", "Read"}."Write" ("step")) -> ("error out"=w110:errorcluster)  [unwired: 7 in, 1 out]
      }
      frame "Exit" {
        n166 = flat-sequence {
          tunnel: w346 -> [w351]
          tunnel: w345 -> [w357]
          frame #0 {
            n167 = call "ExitAllResource.vi"("error in (no error)"=w351) -> ("error out"=w352:errorcluster)  [unwired: 10 in]
            n168 = property class="App"(error in=w352) -> ("App.Kind"=w353:T7)  [unwired: 1 in, 2 out]
            n169 = case shown="\"Run Time System\"" w353 {
              frame "Development System", Default {
              }
              frame "Run Time System" {
                n170 = control-ref of="本VI"() -> (w354:refnum<vi>)
                n171 = invoke class="VI" method="FP.Close"(reference=w354) -> (error out=w355:errorcluster)  [unwired: 2 in, 2 out]
                n172 = call <vilib>:"Clear Errors.vi"("error in (no error)"=w355) -> ()  [unwired: 5 in, 2 out]
              }
            }
          }
          frame #1 {
            n173 = disable-structure shown="禁用" {
              frame Disabled {
                n174 = Quit LabVIEW(quit? (T)=TRUE) -> ()
              }
              frame Enabled {
              }
            }
            n175 = Unbundle By Name(w357) -> ("MainVI"=w356:refnum<vi>)
            n176 = Close Reference(reference=w356) -> ()  [unwired: 1 in, 1 out]
          }
        }
        n177 = call "AMC Destroy Message Queue.vi"("error in (no error)"=w346, "Message Queue in"=w348) -> ("error out"=w347:errorcluster)  [unwired: 9 out]
      }
    }
  }
  n178 = case shown="真" FALSE {
    frame False {
    }
    frame True {
      n179 = call "IO.vi"("DO DATA"=bool[] [FALSE, FALSE, FALSE], "IO Name"=string[] ["Green", "Red", "Yellow"], "IO?"=enum16{"DI", "DO"}."DO") -> ()  [unwired: 6 in, 3 out]
    }
  }
